vi "Compare Image Sizes.vi"(8 "error in (no error)":errorcluster, 9 "Image Refnum 2":T1, 11 "Image Refnum 1":T1) -> (0 "error out":errorcluster, 1 "Image Refnum 2 (dup)":T1, 3 "Image Refnum 1 (dup)":T1, 4 "Comparable Images?":bool)   [LabVIEW 2021, in "Image.lvlib"]
uses:
  <vilib>/vision/Image Controls.llb/IMAQ Image.ctl
  Image.lvlib
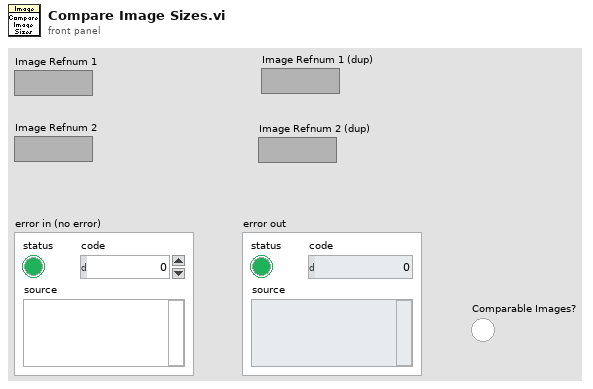
[diagram p1: front panel]
types:
  T1 = typedef "IMAQ Image.ctl" = refnum<image>
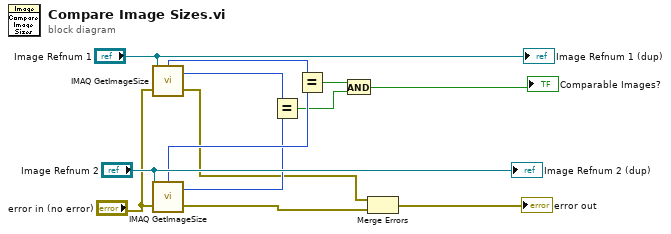
[diagram p0: block diagram]
diagram:
  n1 = call "IMAQ GetImageSize"("Image"="Image Refnum 1", "error in (no error)"="error in (no error)") -> ("Y Resolution"=w8:i32, "X Resolution"=w10:i32, "error out"=w5:errorcluster)  [unwired: 2 in]
  n2 = call "IMAQ GetImageSize"("Image"="Image Refnum 2", "error in (no error)"="error in (no error)") -> ("Y Resolution"=w7:i32, "X Resolution"=w9:i32, "error out"=w6:errorcluster)  [unwired: 2 in]
  n3 = Equal?(x=w8, y=w7) -> (x = y?=w2:bool)
  n4 = Equal?(x=w10, y=w9) -> (x = y?=w3:bool)
  n5 = And(x=w3, y=w2) -> (x .and. y?=→"Comparable Images?":bool)
  n6 = Merge Errors(w5, w6) -> (→"error out":errorcluster)
  "Image Refnum 2 (dup)" <- "Image Refnum 2"
  "Image Refnum 1 (dup)" <- "Image Refnum 1"
